vi "Dmux.vi"(0 "in":bool, 2 "sel":bool) -> (4 "a":bool, 5 "b":bool)   [LabVIEW 2014]
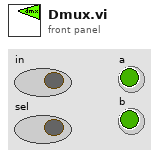
[diagram p1: front panel]
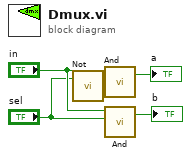
[diagram p0: block diagram]
diagram:
  n1 = call "Not.vi"("in"="sel") -> ("out"=w5:bool)  [unwired: 2 in]
  n2 = call "And.vi"("b"=w5, "a"="in") -> ("out"=→"a":bool)  [unwired: 3 in]
  n3 = call "And.vi"("b"="sel", "a"="in") -> ("out"=→"b":bool)  [unwired: 3 in]
